vi "Get Path Regex.vi"(8 "error in (no error)":errorcluster, 11 "Test WebSocket Page Controller in":refnum<class "Test WebSocket Page Controller.lvclass">) -> (0 "error out":errorcluster, 2 "Path Regex":string, 3 "Test WebSocket Page Controller out":refnum<class "Test WebSocket Page Controller.lvclass">)   [LabVIEW 2020, in "Test WebSocket Page Controller.lvclass"]
uses:
  Test WebSocket Page Controller.lvclass
  Test WebSocket Page Controller.lvclass/Test WebSocket Page Controller.ctl
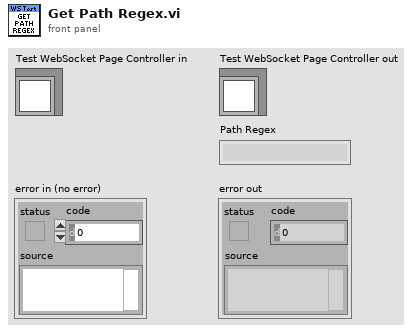
[diagram p1: front panel]
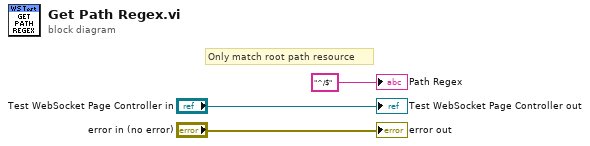
[diagram p0: block diagram]
diagram:
  # "Only match root path resource"
  "error out" <- "error in (no error)"
  "Test WebSocket Page Controller out" <- "Test WebSocket Page Controller in"
  "Path Regex" <- "^/$" ("Path Regex")
